vi "INI File Path FGV.vi"(8 "error in (no error)":errorcluster, 11 "Action":enum16{"Get", "Init"}(ring)) -> (0 "error out":errorcluster, 3 "Path":path)   [LabVIEW 2016, in "System Mapping Tool.lvlib"]
uses:
  System Mapping Tool.lvlib
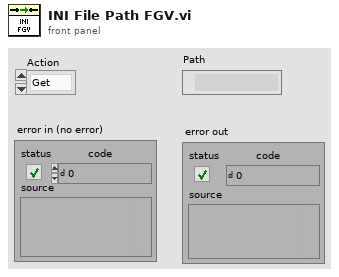
[diagram p1: front panel]
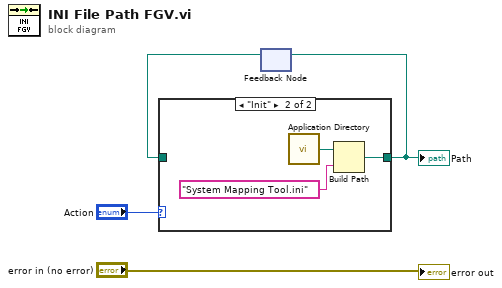
[diagram p0: block diagram]
diagram:
  n1 = feedback #1() -> (w2:path)  [unwired: 1 in]
  n2 = case shown="\"Init\"" "Action" {
    tunnel: [w5 w8] -> w3
    tunnel: w2 -> [w5 _]
    frame "Get", Default {
    }
    frame "Init" {
      n3 = call <vilib>:"Application Directory.vi"() -> ("Application Directory"=w7:path)
      n4 = Build Path(base path=w7, name or relative path="System Mapping Tool.ini") -> (appended path=w8:path)
    }
  }
  "Path" <- w3
  n5 = feedback-in #1(w3) -> ()
  "error out" <- "error in (no error)"
